vi "Z_norm_to_um_scaling_linearFit.vi"(0 "Input Array(Znorm, Z_um)":dbl[][](array[numeric]), 3 "error in (no error)":errorcluster) -> (7 "Znorm_to_um_scaling":dbl, 10 "error out":errorcluster)   [LabVIEW 2020]
uses:
  Globals/gl_Calibration globals.vi
  <vilib>/Analysis/NI_AALPro.lvlib
panel:
  out "Linear Model Graph":dbl[][](graph)
  out "intercept":dbl
  out "slope":dbl
  out "Best Linear Fit":dbl[](array[numeric])
  out "Intercept":dbl
  out "best fit":dynamicdata(graph)
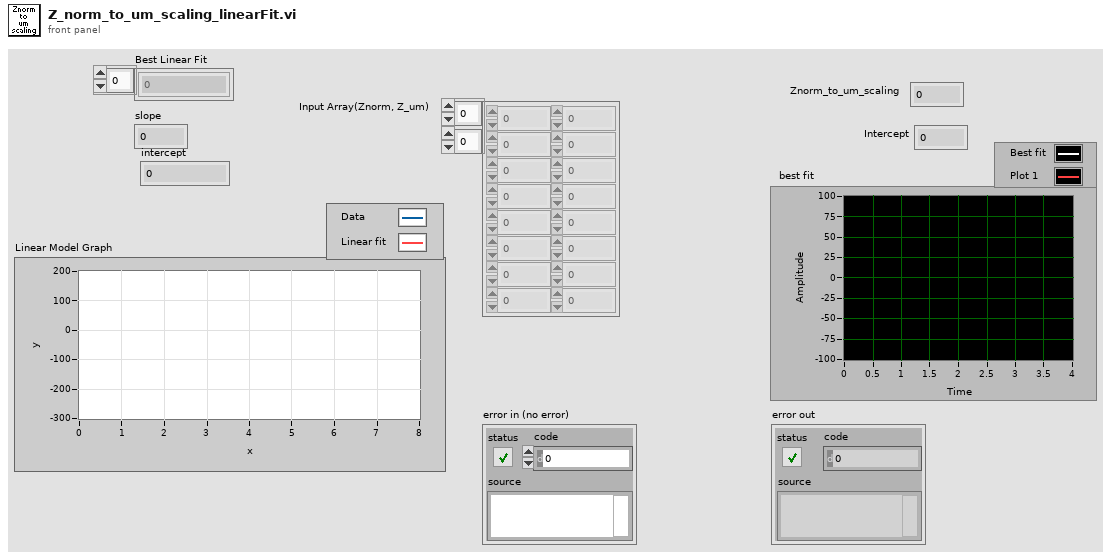
[diagram p1: front panel]
types:
  T1 = typedef "General Scan Parameters.ctl" = cluster{"Field of View":sgl, "Frame Size":u16, "Dwell Time (ms)":dbl, "Wavelength (nm)":dbl, "Zoom":dbl, "AOL Xc":sgl, "AOL Yc":sgl, "AOL Zc":sgl, "AOL Mode":enum16{"Raster", "Structural", "Pointing", "Mini Scan", "Alignment"}, "Imaging Mode":enum16{"Live Imaging", "AOL Zstack", "Motor Zstack", "Functional Imaging"}}
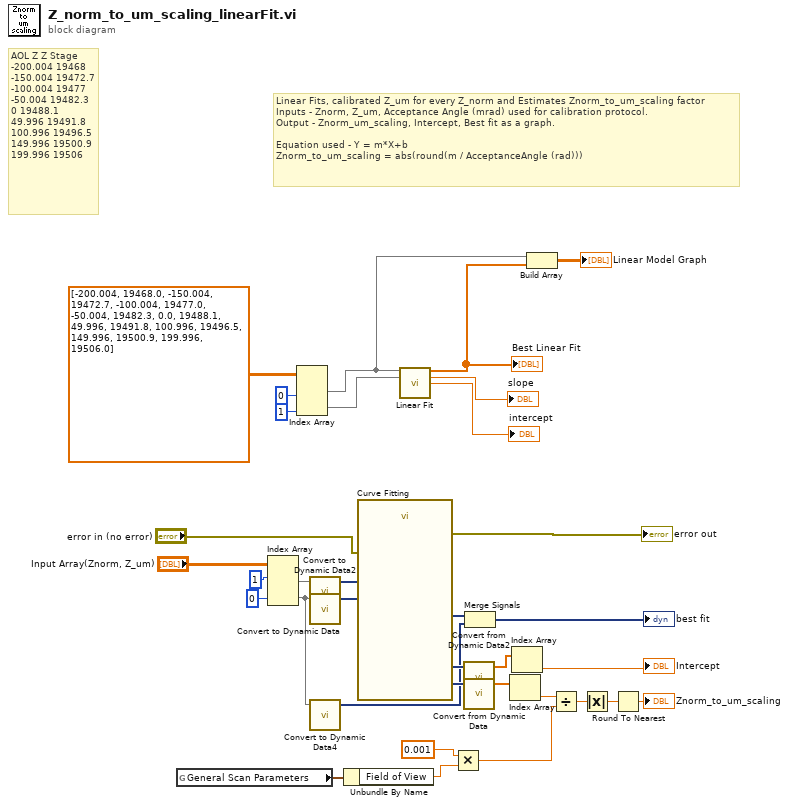
[diagram p0: block diagram]
diagram:
  # "AOL Z\tZ Stage\n-200.004\t19468\n-150.004\t19472.7\n-100.004\t19477\n-50.004\t19482.3\n0\t19488.1\n49.996\t19491.8\n100.996\t19496.5\n149.996\t19500.9\n199.996\t19506"
  # "Linear Fits, calibrated Z_um for every Z_norm and Estimates Znorm_to_um_scaling factor\nInputs - Znorm, Z_um, Acceptance Angle (mrad) used for calibration protocol.\nOutput - Znorm_um_scaling, Intercept, Best fit as a graph.\n\nEquation used - Y = m*X+b\nZnorm_to_um_scaling = abs(round(m / AcceptanceAngle (rad)))"
  n1 = global read "gl_Calibration globals.vi" "General Scan Parameters"() -> (w14:T1)
  n2 = Index Array(array="Input Array(Znorm, Z_um)", index (row) #1=1 ("disabled index (col)"), index (row) #2=0 ("index (row)")) -> (element #1=w24:dbl[], element #2=w25:dbl[])  [unwired: 2 in]
  n3 = Index Array(array=dbl[][] [[-200.004, 19468.0], [-150.004, 19472.7], [-100.004, 19477.0], [-50.004, 19482.3], [0.0, 19488.1], [49.996, 19491.8], [100.996, 19496.5], [149.996, 19500.9], [199.996, 19506.0]] ("Input Array(Znorm, Z_um)"), index (col) #1=0 ("disabled index (col)"), index (col) #2=1 ("index (col)")) -> (element #1=w2:dbl[], element #2=w6:dbl[])  [unwired: 2 in]
  n4 = call "Convert to Dynamic Data2"("Array"=w24) -> ("Dynamic Data Type"=w17:dynamicdata)  [unwired: 3 in]
  n5 = call "Convert to Dynamic Data"("Array"=w25) -> ("Dynamic Data Type"=w18:dynamicdata)  [unwired: 3 in]
  n6 = call "Convert to Dynamic Data4"("Array"=w25) -> ("Dynamic Data Type"=w22:dynamicdata)  [unwired: 3 in]
  n7 = Unbundle By Name(w14) -> ("Field of View"=w13:sgl)
  n8 = call "Curve Fitting"("error in (no error)"="error in (no error)", "Locations"=w18, "Signals"=w17) -> ("error out"=→"error out":errorcluster, "best fit"=w23:dynamicdata, "slope"=w34:dynamicdata, "intercept"=w32:dynamicdata)  [unwired: 3 in, 2 out]
  n9 = call <vilib>:"Linear Fit.vi"("Y"=w2, "X"=w6) -> ("Best Linear Fit"=w1:dbl[], "slope"=→"slope":dbl, "intercept"=→"intercept":dbl)  [unwired: 9 in, 2 out]
  "Best Linear Fit" <- w1
  n10 = Multiply(x=0.001, y=w13) -> (x*y=w27:dbl)
  n11 = call "Convert from Dynamic Data2"("Dynamic Data Type"=w32) -> ("Array"=w21:dbl[])  [unwired: 3 in]
  n12 = call "Convert from Dynamic Data"("Dynamic Data Type"=w34) -> ("Array"=w33:dbl[])  [unwired: 3 in]
  n13 = Merge Signals(w23, w22) -> (→"best fit":dynamicdata)
  n14 = Index Array(array=w33) -> (element=w31:dbl)  [unwired: 1 in]
  n15 = Index Array(array=w21) -> (element=→"Intercept":dbl)  [unwired: 1 in]
  n16 = Build Array(w2, w1) -> (→"Linear Model Graph":dbl[][])
  n17 = Divide(x=w31, y=w27) -> (x/y=w30:dbl)
  n18 = Absolute Value(x=w30) -> (abs(x)=w29:dbl)
  n19 = Round To Nearest(number=w29) -> (nearest integer value=→"Znorm_to_um_scaling":dbl)
